vi "Pick up Item.vi"(8 "error in (no error)":errorcluster, 10 "Beverage.lvclass":refnum<class "Beverage.lvclass">, 11 "Customer in":refnum<class "Customer.lvclass">) -> (0 "error out":errorcluster, 3 "Customer out":refnum<class "Customer.lvclass">)   [LabVIEW 2023, in "Customer.lvlib" / "Customer.lvclass"]
doc: "This function is called when a customer is notified that a drink order has been completed."
uses:
  Customer.lvclass
  Beverages/Beverage/Beverage.lvclass
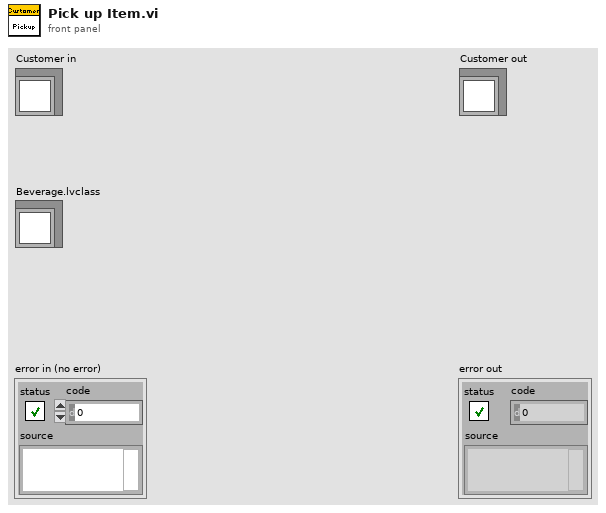
[diagram p1: front panel]
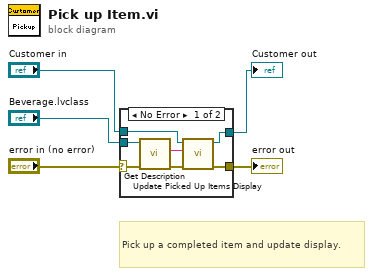
[diagram p0: block diagram]
diagram:
  # "Pick up a completed item and update display."
  n1 = case shown="No Error" "error in (no error)" {
    selector: "error in (no error)" -> [w7 w14]
    tunnel: [w9 w14] -> w4
    tunnel: [w8 w13] -> w2
    tunnel: "Customer in" -> [w12 w13]
    tunnel: "Beverage.lvclass" -> [w11 _]
    frame No Error {
      n2 = call "Get Description.vi"("error in"=w7, "Beverage in"=w11) -> ("error out"=w6:errorcluster, "Description"=w10:string)  [unwired: 7 in, 1 out]
      n3 = call-dynamic "Update Picked Up Items Display.vi"("error in (no error)"=w6, "Item Description"=w10, "Customer in"=w12) -> ("error out"=w9:errorcluster, "Customer out"=w8:refnum<class "Customer.lvclass">)  [unwired: 7 in]
    }
    frame Error {
    }
  }
  "error out" <- w4
  "Customer out" <- w2
